vi "Test_Thresholding_Algorithm.vi"() -> ()   [LabVIEW 2020]
panel:
  out "x/y":dbl
  in  "delta":u16=1 min=1 max=50 step=1
  out "first subarray":u16[](array[numeric])
  out "index of element":i32
  out "output array":u16[](array[numeric])
  out "Image":T1(plugin-control)
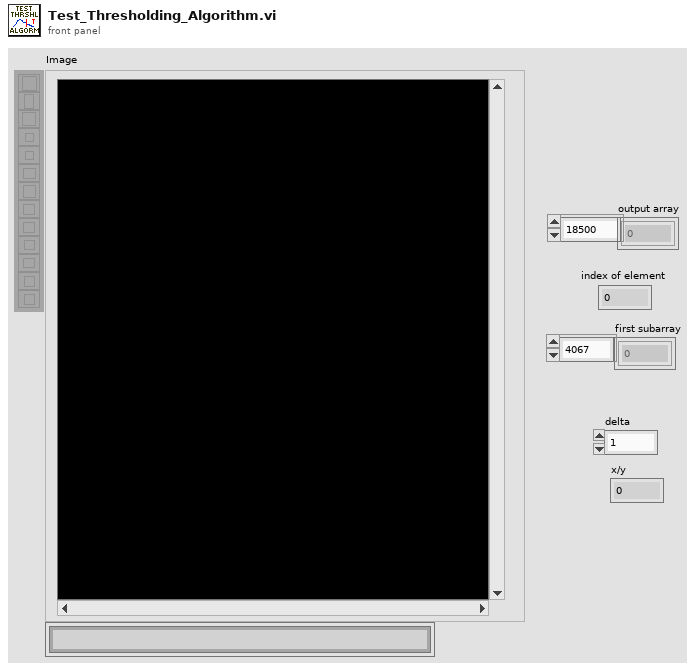
[diagram p1: front panel]
types:
  T1 = typedef "IMAQ Image.ctl" = refnum<image>
  T2 = typedef "Image Type" = u32
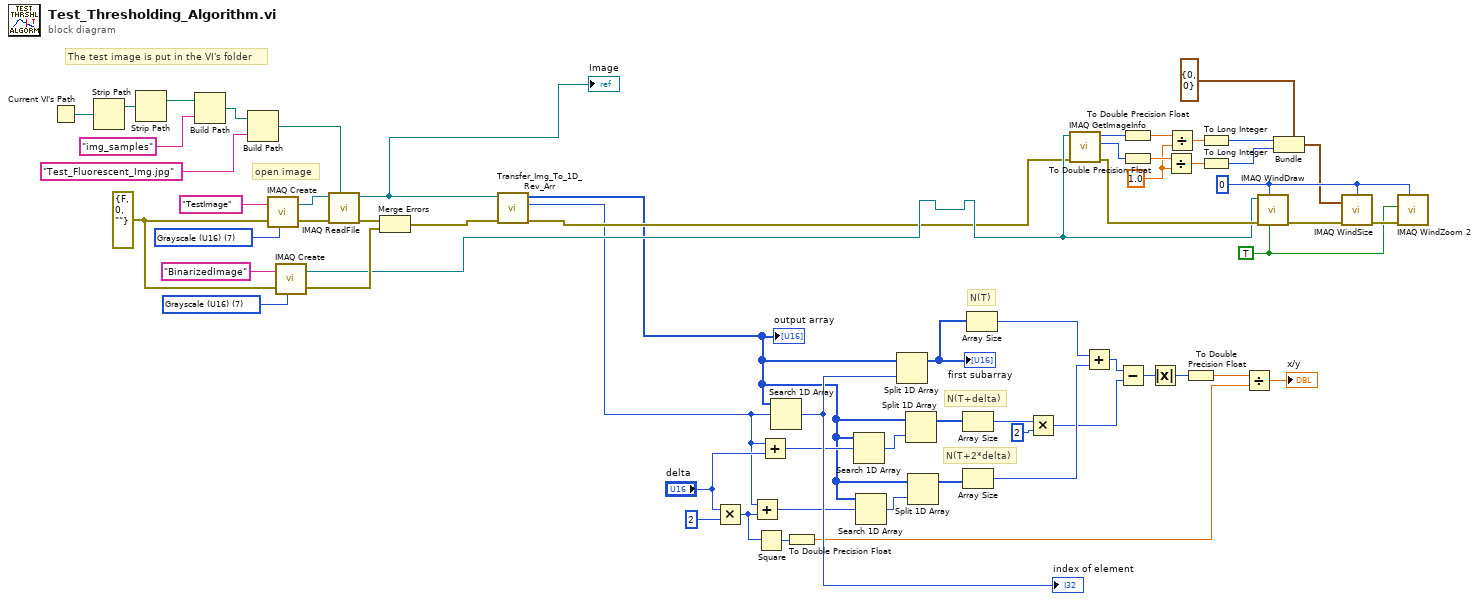
[diagram p0: block diagram]
diagram:
  w38 = 1.0 ("y")
  w37 = TRUE ("Scrollbars? (N)")
  w51 = 0 ("Window Number (0...15)")
  w56 = T2 7 items=["Grayscale (U8)", "Grayscale (I16)", "Grayscale (SGL)", "Complex (CSG)", "RGB (U32)", "HSL (U32)", "RGB (U64)", "Grayscale (U16)"] ("Image Type")
  w60 = T2 7 items=["Grayscale (U8)", "Grayscale (I16)", "Grayscale (SGL)", "Complex (CSG)", "RGB (U32)", "HSL (U32)", "RGB (U64)", "Grayscale (U16)"] ("Image Type")
  w55 = errorcluster {"status"=FALSE, "code"=0, "source"=""} ("error in (no error)")
  # "N(T+2*delta)"
  # "N(T+delta)"
  # "N(T)"
  # "open image"
  # "The test image is put in the VI's folder"
  n1 = Current VI's Path() -> (path=w36:path)
  n2 = Strip Path(path=w36) -> (stripped path=w35:path)  [unwired: 1 out]
  n3 = Strip Path(path=w35) -> (stripped path=w34:path)  [unwired: 1 out]
  n4 = Build Path(base path=w34, name or relative path="img_samples") -> (appended path=w32:path)
  n5 = Build Path(base path=w32, name or relative path="Test_Fluorescent_Img.jpg") -> (appended path=w30:path)
  n6 = call "IMAQ Create"("Image Name"="TestImage", "Image Type"=w60, "error in (no error)"=w55) -> ("New Image"=w58:T1, "error out"=w59:errorcluster)  [unwired: 2 in]
  n7 = call "IMAQ Create"("Image Name"="BinarizedImage", "Image Type"=w56, "error in (no error)"=w55) -> ("New Image"=w6:T1, "error out"=w53:errorcluster)  [unwired: 2 in]
  n8 = call "IMAQ ReadFile"("File Path"=w30, "error in (no error)"=w59, "Image"=w58) -> ("error out"=w54:errorcluster, "Image Out"=w4:T1)  [unwired: 4 in, 3 out]
  "Image" <- w4
  n9 = Merge Errors(w54, w53) -> (w5:errorcluster)
  n10 = call "Transfer_Img_To_1D_Rev_Arr.vi"("error in"=w5, "[IN] Original Image"=w4) -> ("error out"=w3:errorcluster, "[OUT] Threshold Initial"=w1:u16, "[OUT] 1D Sort Rever Img"=w2:u16[])  [unwired: 7 in]
  "output array" <- w2
  n11 = Multiply(x="delta", y=u16 2) -> (x*y=w18:u16)
  n12 = Add(x=w1, y=w18) -> (x+y=w25:u16)
  n13 = Square(x=w18) -> (x^2=w11:u16)
  n14 = Add(x=w1, y="delta") -> (x+y=w7:u16)
  n15 = Search 1D Array(1D array=w2, element=w1) -> (index of element=w28:i32)  [unwired: 1 in]
  "index of element" <- w28
  n16 = To Double Precision Float(number=w11) -> (double precision float=w9:dbl)
  n17 = Search 1D Array(1D array=w2, element=w7) -> (index of element=w24:i32)  [unwired: 1 in]
  n18 = Search 1D Array(1D array=w2, element=w25) -> (index of element=w22:i32)  [unwired: 1 in]
  n19 = Split 1D Array(array=w2, index=w28) -> (first subarray=w29:u16[])  [unwired: 1 out]
  "first subarray" <- w29
  n20 = Split 1D Array(array=w2, index=w24) -> (first subarray=w23:u16[])  [unwired: 1 out]
  n21 = Split 1D Array(array=w2, index=w22) -> (first subarray=w21:u16[])  [unwired: 1 out]
  n22 = Array Size(array=w23) -> (size(s)=w17:i32)
  n23 = Array Size(array=w21) -> (size(s)=w20:i32)
  n24 = Array Size(array=w29) -> (size(s)=w19:i32)
  n25 = Multiply(x=w17, y=2) -> (x*y=w14:i32)
  n26 = call "IMAQ GetImageInfo"("error in (no error)"=w3, "Image"=w6) -> ("error out"=w42:errorcluster, "Y Resolution"=w45:i32, "X Resolution"=w48:i32)  [unwired: 2 in, 5 out]
  n27 = Add(x=w19, y=w20) -> (x+y=w15:i32)
  n28 = Subtract(x=w15, y=w14) -> (x-y=w13:i32)
  n29 = To Double Precision Float(number=w48) -> (double precision float=w47:dbl)
  n30 = To Double Precision Float(number=w45) -> (double precision float=w44:dbl)
  n31 = Absolute Value(x=w13) -> (abs(x)=w12:i32)
  n32 = Divide(x=w44, y=w38) -> (x/y=w43:dbl)
  n33 = Divide(x=w47, y=w38) -> (x/y=w46:dbl)
  n34 = To Double Precision Float(number=w12) -> (double precision float=w10:dbl)
  n35 = To Long Integer(number=w46) -> (32bit integer=w40:i32)
  n36 = To Long Integer(number=w43) -> (32bit integer=w39:i32)
  n37 = Divide(x=w10, y=w9) -> (x/y=→"x/y":dbl)
  n38 = call "IMAQ WindDraw"("Resize to Image Size? (Y)"=w37, "Window Number (0...15)"=w51, "error in (no error)"=w42, "Image"=w6) -> ("error out"=w52:errorcluster)  [unwired: 6 in, 1 out]
  n39 = Bundle(cluster=cluster{"Width":i32, "Height":i32} {"Width"=0, "Height"=0} ("Width & Height"), "Width"=w40, "Height"=w39) -> (w41:cluster{"Width":i32, "Height":i32})
  n40 = call "IMAQ WindSize"("error in (no error)"=w52, "Width & Height"=w41, "Window Number"=w51) -> ("error out"=w50:errorcluster)  [unwired: 3 in, 2 out]
  n41 = call "IMAQ WindZoom 2"("Window Number (0...15)"=w51, "error in (no error)"=w50, "Zoom to Fit? (False)"=w37) -> ()  [unwired: 5 in, 4 out]
